vi "Proceed.vi"(7 "component is ready (Y)":bool=TRUE, 8 "error in (no error)":errorcluster, 10 "ProceedMessage":refnum<class "ProceedMessage.lvclass">, 11 "DAQOrcaFlash in":refnum<class "DAQOrcaFlash.lvclass">) -> (0 "error out":errorcluster, 2 "all observers are ready?":bool, 3 "DAQOrcaFlash out":refnum<class "DAQOrcaFlash.lvclass">)   [LabVIEW 2012, in "DAQOrcaFlash.lvclass"]
uses:
  DAQOrcaFlash.lvclass
  <vilib>/Distrio/Murmex/ProceedMessage/ProceedMessage.lvclass
  DAQOrcaFlash.lvclass/DAQOrcaFlash.ctl
  <vilib>/Distrio/Murmex/Murmex/Murmex.lvclass
panel:
  # "This method is called when the PROCEED\ntrigger is sent. \n\nOverride this method when your component needs to\nrespond to this trigger. \n\nCall parent for proper implementation"
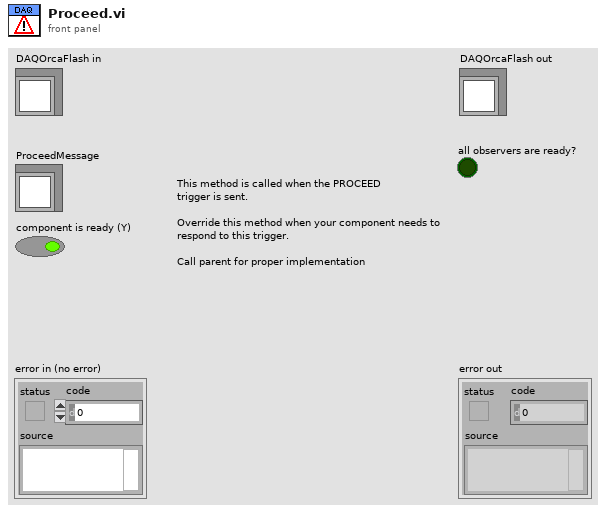
[diagram p1: front panel]
types:
  T1 = typedef "DAQOrcaFlash.lvclass/imaging_mode.ctl" = enum16{"focus mode", "single sweep"}
  T2 = typedef "IMAQ Image.ctl" = refnum<image>
  T3 = cluster{"width":u32, "height":u32, "datatype":u32}
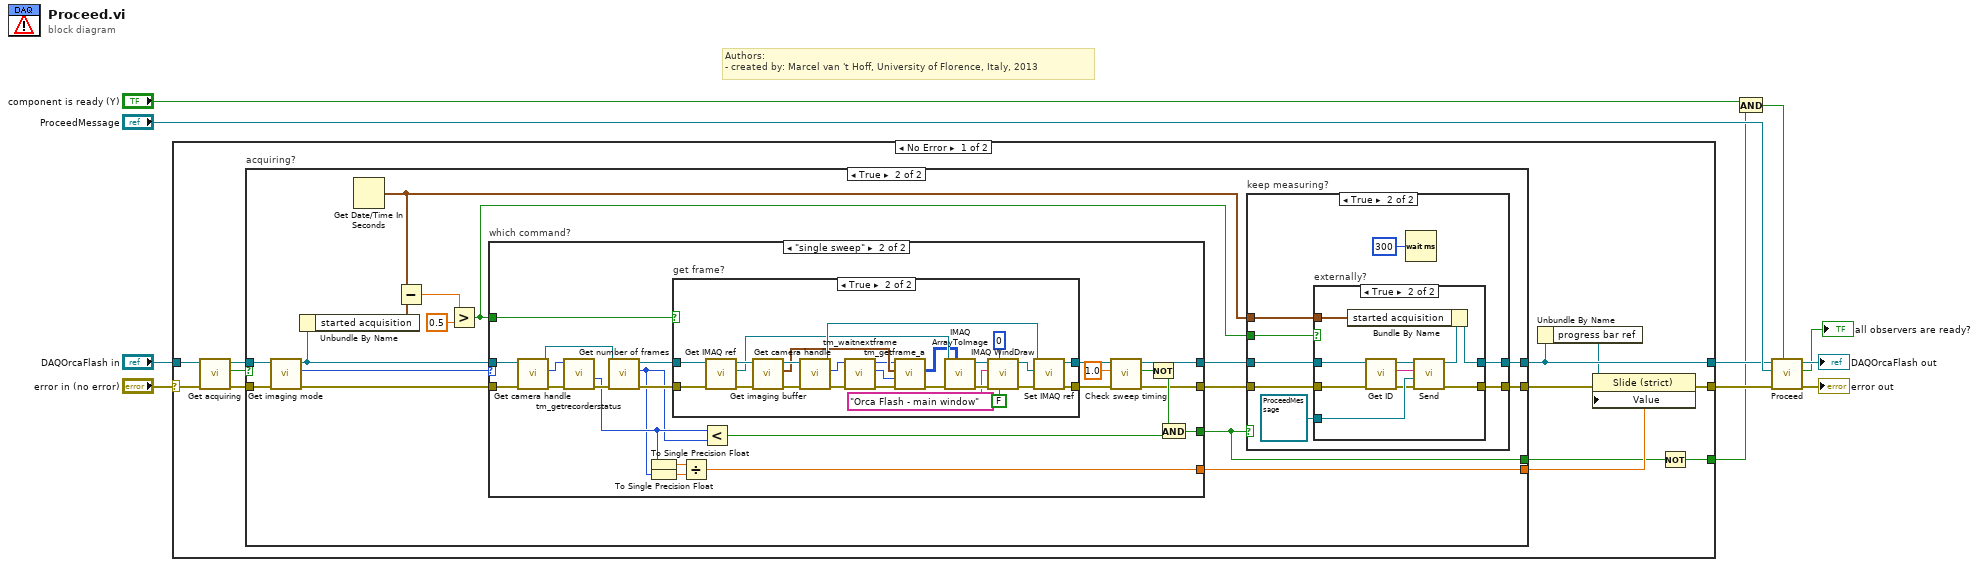
[diagram p0: block diagram]
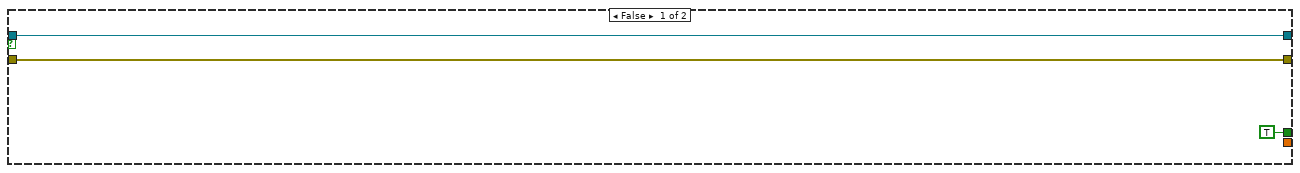
[diagram p2: hidden frame]
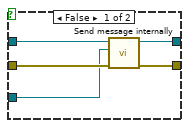
[diagram p4: hidden frame]
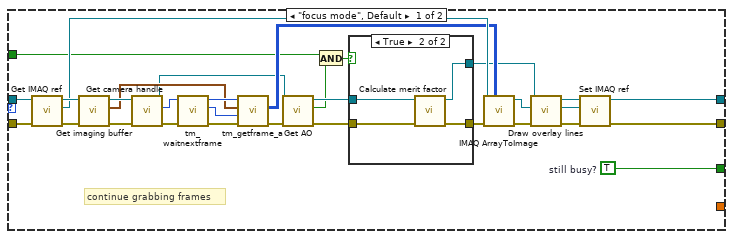
[diagram p5: hidden frame]
diagram:
  # "Authors: \n- created by: Marcel van 't Hoff, University of Florence, Italy, 2013"
  n1 = case shown="No Error" "error in (no error)" {
    selector: "error in (no error)" -> [w21 w156]
    tunnel: [w15 w156] -> w6
    tunnel: [w18 w155] -> w5
    tunnel: "DAQOrcaFlash in" -> [w23 w155]
    tunnel: [w12 _] -> w3
    frame No Error {
      n2 = call "Get acquiring.vi"("error in (no error)"=w21, "DAQMH121119OrcaFlash in"=w23) -> ("error out"=w20:errorcluster, "is acquiring?"=w19:bool, "DAQMH121119OrcaFlash out"=w22:refnum<class "DAQOrcaFlash.lvclass">)  [unwired: 7 in]
      n3 = case "acquiring?" shown="True" w19 {
        tunnel: [w25 w36] -> w14
        tunnel: [w26 w37] -> w18
        tunnel: w22 -> [w26 w40]
        tunnel: w20 -> [w25 w39]
        tunnel: [_ w38] -> w16
        tunnel: [TRUE ("proceed?") w29] -> w13
        frame False {
        }
        frame True {
          n4 = call "Get imaging mode.vi"("error in (no error)"=w39, "DAQMH121119OrcaFlash in"=w40) -> ("error out"=w42:errorcluster, "imaging mode"=w41:T1, "DAQMH121119OrcaFlash out"=w32:refnum<class "DAQOrcaFlash.lvclass">)  [unwired: 7 in]
          n5 = Unbundle By Name(w32) -> ("started acquisition"=w33:timestamp)
          n6 = Get Date/Time In Seconds() -> (seconds since 1Jan1904=w31:timestamp)
          n7 = Subtract(x=w31, y=w33) -> (x-y=w34:dbl)
          n8 = Greater?(x=w34, y=0.5) -> (0:w30:bool)
          n9 = case "which command?" shown="\"single sweep\"" w41 {
            tunnel: w42 -> [w97 w127]
            tunnel: w32 -> [w98 w125]
            tunnel: [w96 w107] -> w27
            tunnel: [w95 w108] -> w28
            tunnel: [_ w117] -> w38
            tunnel: [w94 w105] -> w29
            tunnel: w30 -> [w75 w116]
            frame "focus mode", Default {
              w94 = TRUE  # still busy?
              # "continue grabbing frames"
              n10 = call "Get IMAQ ref.vi"("error in (no error)"=w97, "DAQMH121119OrcaFlash in"=w98) -> ("error out"=w89:errorcluster, "IMAQ reference"=w83:T2, "DAQMH121119OrcaFlash out"=w91:refnum<class "DAQOrcaFlash.lvclass">)  [unwired: 7 in]
              n11 = call "Get imaging buffer.vi"("error in (no error)"=w89, "DAQMH121119OrcaFlash in"=w91) -> ("error out"=w88:errorcluster, "imaging buffer"=w85:T3, "DAQMH121119OrcaFlash out"=w90:refnum<class "DAQOrcaFlash.lvclass">)  [unwired: 5 in, 2 out]
              n12 = call "Get camera handle.vi"("error in (no error)"=w88, "DAQMH121119OrcaFlash in"=w90) -> ("error out"=w92:errorcluster, "cam handle"=w93:u32, "DAQMH121119OrcaFlash out"=w78:refnum<class "DAQOrcaFlash.lvclass">)  [unwired: 7 in]
              n13 = call <userlib>:"tm_waitnextframe.vi"("error in (no error)"=w92, "Handle in"=w93) -> ("error out"=w87:errorcluster, "Frame Index"=w84:i32, "Handle out"=w86:u32)  [unwired: 6 in, 1 out]
              n14 = call <userlib>:"tm_getframe_a.vi"("error in (no error)"=w87, "Frame Index"=w84, "Buffer Info"=w85, "Handle in"=w86) -> ("error out"=w80:errorcluster, "Data 16"=w81:u16[][])  [unwired: 3 in, 3 out]
              n15 = call-dynamic "Get AO.vi"("error in (no error)"=w80, "DAQOrcaFlash in"=w78) -> ("error out"=w79:errorcluster, "AO"=w76:bool, "DAQOrcaFlash out"=w77:refnum<class "DAQOrcaFlash.lvclass">)  [unwired: 7 in]
              n16 = And(x=w75, y=w76) -> (x .and. y?=w74:bool)
              n17 = case shown="True" w74 {
                tunnel: [w100 w104] -> w82
                tunnel: w79 -> [w100 w101]
                tunnel: w77 -> [w99 w102]
                tunnel: [w99 w103] -> w68
                frame False {
                }
                frame True {
                  n18 = call-dynamic "Calculate merit factor.vi"("error in (no error)"=w101, "DAQOrcaFlash in"=w102) -> ("error out"=w104:errorcluster, "DAQOrcaFlash out"=w103:refnum<class "DAQOrcaFlash.lvclass">)  [unwired: 8 in]
                }
              }
              n19 = call "IMAQ ArrayToImage"("Image Pixels (U16)"=w81, "error in (no error)"=w82, "Image"=w83) -> ("error out"=w73:errorcluster, "Image Out"=w71:T2)  [unwired: 7 in]
              n20 = call "Draw overlay lines.vi"("error in (no error)"=w73, "IMAQ reference"=w71, "DAQOrcaFlash in"=w68) -> ("error out"=w72:errorcluster, "IMAQ reference out"=w70:T2, "DAQOrcaFlash out"=w69:refnum<class "DAQOrcaFlash.lvclass">)  [unwired: 6 in]
              n21 = call "Set IMAQ ref.vi"("error in (no error)"=w72, "IMAQ reference"=w70, "DAQMH121119OrcaFlash in"=w69) -> ("error out"=w96:errorcluster, "DAQMH121119OrcaFlash out"=w95:refnum<class "DAQOrcaFlash.lvclass">)  [unwired: 7 in]
            }
            frame "single sweep" {
              n22 = call "Get camera handle.vi"("error in (no error)"=w127, "DAQMH121119OrcaFlash in"=w125) -> ("error out"=w126:errorcluster, "cam handle"=w124:u32, "DAQMH121119OrcaFlash out"=w123:refnum<class "DAQOrcaFlash.lvclass">)  [unwired: 7 in]
              n23 = call <userlib>:"tm_getrecorderstatus.vi"("error in (no error)"=w126, "Handle"=w124) -> ("error out"=w122:errorcluster, "Count"=w115:i32)  [unwired: 6 in, 2 out]
              n24 = call "Get number of frames.vi"("error in (no error)"=w122, "DAQMH121119OrcaFlash in"=w123) -> ("error out"=w121:errorcluster, "no. of frames"=w114:i32, "DAQMH121119OrcaFlash out"=w120:refnum<class "DAQOrcaFlash.lvclass">)  [unwired: 7 in]
              n25 = To Single Precision Float(number=w115) -> (single precision float=w118:sgl)
              n26 = To Single Precision Float(number=w114) -> (single precision float=w119:sgl)
              n27 = case "get frame?" shown="True" w116 {
                tunnel: w121 -> [w129 w146]
                tunnel: w120 -> [w128 w145]
                tunnel: [w128 w143] -> w110
                tunnel: [w129 w144] -> w109
                frame False {
                }
                frame True {
                  n28 = call "Get IMAQ ref.vi"("error in (no error)"=w146, "DAQMH121119OrcaFlash in"=w145) -> ("error out"=w153:errorcluster, "IMAQ reference"=w148:T2, "DAQMH121119OrcaFlash out"=w150:refnum<class "DAQOrcaFlash.lvclass">)  [unwired: 7 in]
                  n29 = call "Get imaging buffer.vi"("error in (no error)"=w153, "DAQMH121119OrcaFlash in"=w150) -> ("error out"=w154:errorcluster, "imaging buffer"=w142:T3, "DAQMH121119OrcaFlash out"=w152:refnum<class "DAQOrcaFlash.lvclass">)  [unwired: 5 in, 2 out]
                  n30 = call "Get camera handle.vi"("error in (no error)"=w154, "DAQMH121119OrcaFlash in"=w152) -> ("error out"=w138:errorcluster, "cam handle"=w141:u32, "DAQMH121119OrcaFlash out"=w151:refnum<class "DAQOrcaFlash.lvclass">)  [unwired: 7 in]
                  n31 = call <userlib>:"tm_waitnextframe.vi"("error in (no error)"=w138, "Handle in"=w141) -> ("error out"=w137:errorcluster, "Frame Index"=w139:i32, "Handle out"=w140:u32)  [unwired: 6 in, 1 out]
                  n32 = call <userlib>:"tm_getframe_a.vi"("error in (no error)"=w137, "Frame Index"=w139, "Buffer Info"=w142, "Handle in"=w140) -> ("error out"=w149:errorcluster, "Data 16"=w147:u16[][])  [unwired: 3 in, 3 out]
                  n33 = call "IMAQ ArrayToImage"("Image Pixels (U16)"=w147, "error in (no error)"=w149, "Image"=w148) -> ("error out"=w136:errorcluster, "Image Out"=w134:T2)  [unwired: 7 in]
                  n34 = call "IMAQ WindDraw"("Resize to Image Size? (Y)"=FALSE, "Window Number (0...15)"=0, "error in (no error)"=w136, "Title"="Orca Flash - main window", "Image"=w134) -> ("error out"=w135:errorcluster, "Image Out (duplicate)"=w133:T2)  [unwired: 5 in]
                  n35 = call "Set IMAQ ref.vi"("error in (no error)"=w135, "IMAQ reference"=w133, "DAQMH121119OrcaFlash in"=w151) -> ("error out"=w144:errorcluster, "DAQMH121119OrcaFlash out"=w143:refnum<class "DAQOrcaFlash.lvclass">)  [unwired: 7 in]
                }
              }
              n36 = Divide(x=w118, y=w119) -> (x/y=w117:sgl)
              n37 = Less?(x=w115, y=w114) -> (x < y?=w106:bool)
              n38 = call-dynamic "Check sweep timing.vi"("error in (no error)"=w109, "Tolerance (s)"=1.0, "DAQOrcaFlash in"=w110) -> ("error out"=w107:errorcluster, "out of time?"=w112:bool, "DAQOrcaFlash out"=w108:refnum<class "DAQOrcaFlash.lvclass">)  [unwired: 6 in]
              n39 = Not(x=w112) -> (.not. x?=w111:bool)
              n40 = And(x=w111, y=w106) -> (x .and. y?=w105:bool)
            }
          }
          n41 = case "keep measuring?" shown="True" w29 {
            tunnel: w27 -> [w43 w47]
            tunnel: [w43 w50] -> w36
            tunnel: w28 -> [w44 w52]
            tunnel: [w44 w51] -> w37
            tunnel: w30 -> [_ w49]
            tunnel: w31 -> [_ w48]
            frame False {
            }
            frame True {
              n42 = case "externally?" shown="True" w49 {
                tunnel: w47 -> [w57 w63]
                tunnel: refnum<class "ProceedMessage.lvclass"> refnum ("ProceedMessage") -> [w56 w65]
                tunnel: w52 -> [w55 w66]
                tunnel: [w54 w58] -> w51
                tunnel: [w53 w67] -> w50
                tunnel: w48 -> [_ w60]
                frame False {
                  n43 = call <vilib>:"Send message internally.vi"("error in (no error)"=w57, "Message"=w56, "Murmex in"=w55) -> ("error out"=w53:errorcluster, "Murmex out"=w54:refnum<class "DAQOrcaFlash.lvclass">)  [unwired: 7 in]
                }
                frame True {
                  n44 = call <vilib>:"Get ID.vi"("error in (no error)"=w63, "Murmex in"=w66) -> ("error out"=w62:errorcluster, "component id"=w61:string, "Murmex out"=w64:refnum<class "DAQOrcaFlash.lvclass">)  [unwired: 7 in]
                  n45 = call <vilib>:"Send.vi"("error in (no error)"=w62, "Message"=w65, "recipient"=w61, "Murmex in"=w64) -> ("error out"=w67:errorcluster, "Murmex out"=w59:refnum<class "DAQOrcaFlash.lvclass">)  [unwired: 6 in]
                  n46 = Bundle By Name(cluster=w59, "started acquisition"=w60) -> (w58:refnum<class "DAQOrcaFlash.lvclass">)
                }
              }
              n47 = Wait (ms)(milliseconds to wait=u32 300) -> ()  [unwired: 1 out]
            }
          }
        }
      }
      n48 = Unbundle By Name(w18) -> ("progress bar ref"=w17:refnum<vi>)
      n49 = property class="Slide (strict)"(reference=w17, error in=w14, "Value"=w16) -> (error out=w15:errorcluster)  [unwired: 1 out]
      n50 = Not(x=w13) -> (.not. x?=w12:bool)
    }
    frame Error {
    }
  }
  n51 = And(x="component is ready (Y)", y=w3) -> (x .and. y?=w2:bool)
  n52 = call-parent "Proceed.vi"("component is ready (Y)"=w2, "error in (no error)"=w6, "ProceedMessage"="ProceedMessage", "Murmex in"=w5) -> ("error out"=→"error out":errorcluster, "all observers are ready?"=→"all observers are ready?":bool, "Murmex out"=→"DAQOrcaFlash out":refnum<class "DAQOrcaFlash.lvclass">)  [unwired: 5 in]
